vi "Forward Simulation Object.vi"(1 "Time step":dbl, 2 "Global Acceleration in":refnum<class "Vector2.lvclass">, 3 "Simulation Object in":refnum<class "SimulationObject.lvclass">) -> (0 "Simulation Object out":refnum<class "SimulationObject.lvclass">)   [LabVIEW 2022 SP3, in "PhysicsSystem.lvclass"]
uses:
  PhysicsSystem.lvclass
  Objects/SimulationObject/SimulationObject.lvclass
  Math/Vector2/Vector2.lvclass
  Objects/SimulationObject/SimulationObject.lvclass/SimulationObject.ctl
  Objects/Components/Transform/Transform.lvclass/Transform.ctl
  Objects/Components/PhysicsComponent/PhysicsComponent.lvclass/PhysicsComponent.ctl
  Objects/Components/PhysicsComponent/PhysicsComponent.lvclass
  Objects/Components/Transform/Transform.lvclass
  PhysicsSystem.lvclass/PhysicsSystem.ctl
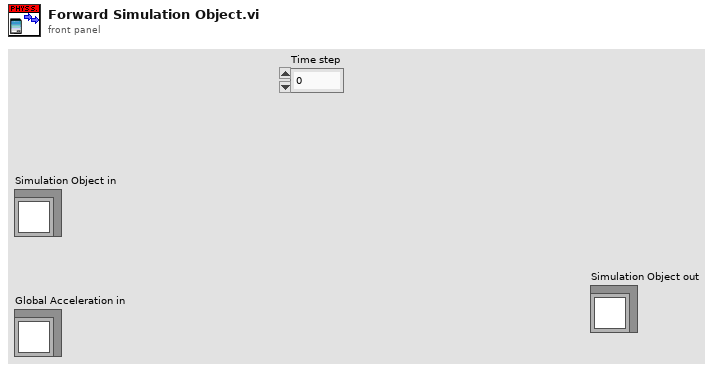
[diagram p1: front panel]
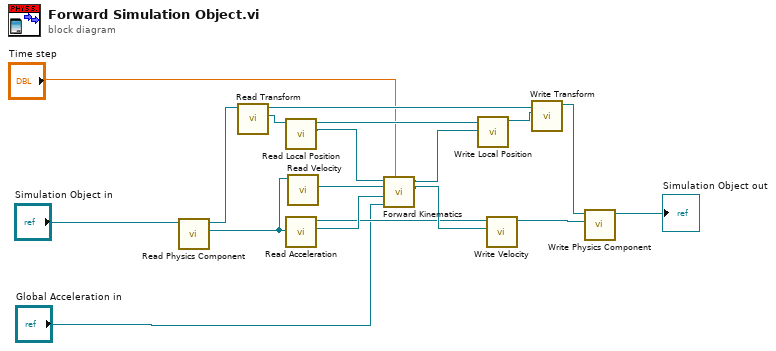
[diagram p0: block diagram]
diagram:
  n1 = call "Read Physics Component.vi"("SimulationObject in"="Simulation Object in") -> ("PhysicsComponent.lvclass"=w12:refnum<class "PhysicsComponent.lvclass">, "SimulationObject out"=w18:refnum<class "SimulationObject.lvclass">)  [unwired: 8 in, 1 out]
  n2 = call "Read Transform.vi"("SimulationObject in"=w18) -> ("Transform out"=w16:refnum<class "Transform.lvclass">, "SimulationObject out"=w17:refnum<class "SimulationObject.lvclass">)  [unwired: 8 in, 1 out]
  n3 = call "Read Local Position.vi"("Transform in"=w16) -> ("Local Position out"=w9:refnum<class "Vector2.lvclass">, "Transform out"=w7:refnum<class "Transform.lvclass">)  [unwired: 8 in, 1 out]
  n4 = call "Read Acceleration.vi"("PhysicsComponent in"=w12) -> ("Acceleration out"=w11:refnum<class "Vector2.lvclass">, "PhysicsComponent out"=w5:refnum<class "PhysicsComponent.lvclass">)  [unwired: 8 in, 1 out]
  n5 = call "Read Velocity.vi"("PhysicsComponent in"=w12) -> ("Velocity out"=w10:refnum<class "Vector2.lvclass">)  [unwired: 8 in, 2 out]
  n6 = call "Forward Kinematics.vi"("Time step"="Time step", "Global acceleration in"="Global Acceleration in", "Acceleration in"=w11, "Velocity in"=w10, "Position in"=w9) -> ("Velocity out"=w6:refnum<class "Vector2.lvclass">, "Position out"=w8:refnum<class "Vector2.lvclass">)  [unwired: 2 out]
  n7 = call "Write Local Position.vi"("Local Position in"=w8, "Transform in"=w7) -> ("Transform out"=w15:refnum<class "Transform.lvclass">)  [unwired: 8 in, 1 out]
  n8 = call "Write Velocity.vi"("Velocity in"=w6, "PhysicsComponent in"=w5) -> ("PhysicsComponent out"=w13:refnum<class "PhysicsComponent.lvclass">)  [unwired: 8 in, 1 out]
  n9 = call "Write Transform.vi"("Transform.lvclass"=w15, "SimulationObject in"=w17) -> ("SimulationObject out"=w14:refnum<class "SimulationObject.lvclass">)  [unwired: 8 in, 1 out]
  n10 = call "Write Physics Component.vi"("PhysicsComponent.lvclass"=w13, "SimulationObject in"=w14) -> ("SimulationObject out"=→"Simulation Object out":refnum<class "SimulationObject.lvclass">)  [unwired: 8 in, 1 out]
